vi "Save Axis.vi"(8 "err in":errorcluster caption="エラー入力（エラーなし）", 11 "WaveformGraph入力":refnum<vi>) -> (0 "err out":errorcluster caption="エラー出力")   [LabVIEW 2014]
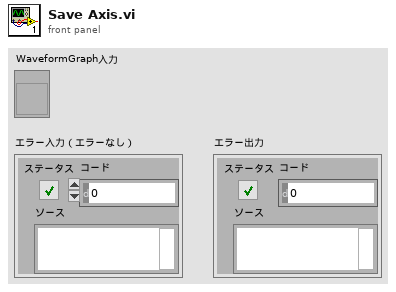
[diagram p1: front panel]
types:
  T1 = typedef "LVRangeTypeDef.ctl" = cluster{"Minimum":dbl, "Maximum":dbl, "Increment":dbl, "Minor Increment":dbl, "Start":dbl}
  T2 = cluster{"NameLbl.Text":string, "UnitLabel.Text":string, "Range":T1}
  T3 = cluster{cluster{"NameLbl.Text":string, "UnitLabel.Text":string, "Range":T1}[], cluster{"NameLbl.Text":string, "UnitLabel.Text":string, "Range":T1}[]}
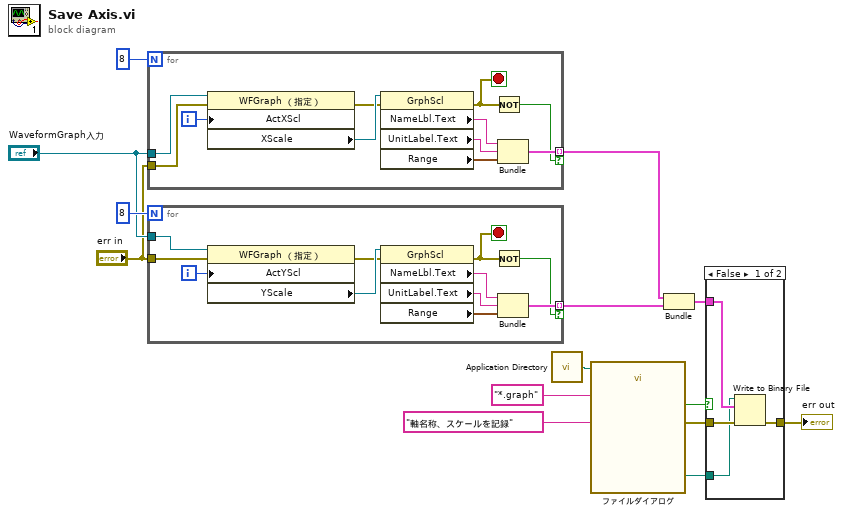
[diagram p0: block diagram]
diagram:
  n1 = for {
    N: 8 -> [_]
    tunnel: "err in" -> [w25]
    tunnel: "WaveformGraph入力" -> [w23]
    tunnel: [w19] -> w2 mode=indexing if=w16
    i -> [w18]
    stop <- w15 stop-if-true
    n2 = property class="WFGraph （指定）"(reference=w23, error in=w25, "ActXScl"=w18) -> (error out=w17:errorcluster, "XScale"=w24:refnum<vi>)  [unwired: 1 out]
    n3 = property class="GrphScl"(reference=w24, error in=w17) -> (error out=w15:errorcluster, "NameLbl.Text"=w22:string, "UnitLabel.Text"=w21:string, "Range"=w20:T1)  [unwired: 1 out]
    n4 = Not(x=w15) -> (.not. x?=w16:bool)
    n5 = Bundle("NameLbl.Text"=w22, "UnitLabel.Text"=w21, "Range"=w20) -> (w19:T2)  [unwired: 1 in]
  }
  n6 = for {
    N: 8 -> [_]
    tunnel: "err in" -> [w36]
    tunnel: "WaveformGraph入力" -> [w34]
    tunnel: [w30] -> w1 mode=indexing if=w27
    i -> [w29]
    stop <- w26 stop-if-true
    n7 = property class="WFGraph （指定）"(reference=w34, error in=w36, "ActYScl"=w29) -> (error out=w28:errorcluster, "YScale"=w35:refnum<vi>)  [unwired: 1 out]
    n8 = property class="GrphScl"(reference=w35, error in=w28) -> (error out=w26:errorcluster, "NameLbl.Text"=w33:string, "UnitLabel.Text"=w32:string, "Range"=w31:T1)  [unwired: 1 out]
    n9 = Not(x=w26) -> (.not. x?=w27:bool)
    n10 = Bundle("NameLbl.Text"=w33, "UnitLabel.Text"=w32, "Range"=w31) -> (w30:T2)  [unwired: 1 in]
  }
  n11 = call <vilib>:"Application Directory.vi"() -> ("Application Directory"=w9:path)
  n12 = call "ファイルダイアログ"("start path"=w9, "prompt"="軸名称、スケールを記録", "pattern (all files)"="*.graph") -> ("selected path"=w3:path, "cancelled"=w5:bool, "error out"=w4:errorcluster)  [unwired: 9 in, 1 out]
  n13 = Bundle(w2, w1) -> (w10:T3)  [unwired: 1 in]
  n14 = case shown="FALSE" w5 {
    tunnel: [w40 w41] -> w14
    tunnel: w10 -> [w39 _]
    tunnel: w4 -> [w38 w41]
    tunnel: w3 -> [w37 _]
    frame False {
      n15 = Write to Binary File(file (use dialog)=w37, data=w39, error in=w38) -> (error out=w40:errorcluster)  [unwired: 3 in, 2 out]
    }
    frame True {
    }
  }
  "err out" <- w14
